vi "__uintGetUint.vi"(8 "Error in (no error)":errorcluster, 11 "UintClass in":refnum<class "UintClass.lvclass">) -> (0 "Error out":errorcluster, 2 "Uint (0)":u8[](array[numeric]), 3 "UintClass out":refnum<class "UintClass.lvclass">)   [LabVIEW 2011, in "UintClass.lvclass"]
uses:
  UintClass.lvclass
  UintClass.lvclass/UintClass.ctl
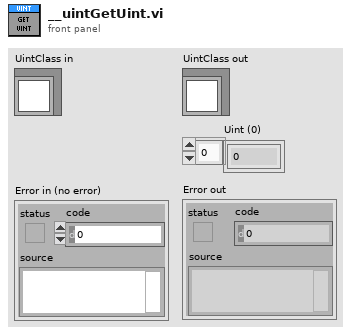
[diagram p1: front panel]
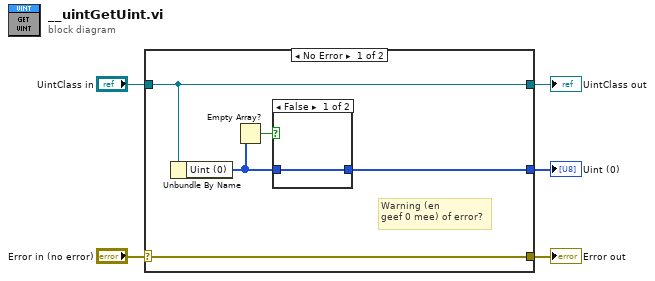
[diagram p0: block diagram]
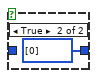
[diagram p2: hidden frame]
diagram:
  n1 = case shown="No Error" "Error in (no error)" {
    selector: "Error in (no error)" -> [w10 w13]
    tunnel: [w10 w13] -> w2
    tunnel: [w9 w14] -> w4
    tunnel: "UintClass in" -> [w9 w14]
    tunnel: [w6 _] -> w3
    frame No Error {
      # "Warning (en\ngeef 0 mee) of error?"
      n2 = Unbundle By Name(w9) -> ("Uint (0)"=w8:u8[])
      n3 = Empty Array?(array=w8) -> (empty?=w7:bool)
      n4 = case shown="False" w7 {
        tunnel: w8 -> [w11 _]
        tunnel: [w11 u8[] [0] ("Uint (0)")] -> w6
        frame False {
        }
        frame True {
        }
      }
    }
    frame Error {
    }
  }
  "UintClass out" <- w4
  "Uint (0)" <- w3
  "Error out" <- w2
